vi "Write.vi"(8 "error in":errorcluster, 10 "CAN Message":T1 {"MSG type" format="%x"; "ID" format="%.0x"}, 11 "PCAN in":refnum<class "PCAN.lvclass">) -> (0 "error out":errorcluster, 3 "PCAN out":refnum<class "PCAN.lvclass">)   [LabVIEW 2025]
uses:
  PCAN.lvclass/PCAN.ctl
  D:/git/HAL/HAL/Configurations/CFG Base/CFG Base.lvclass
  PCAN.lvclass
  C:/Users/tupp_js/Documents/LabVIEW Data/HAL/source/Devices/PCAN/PCAN.lvclass
  C:/Users/tupp_js/Documents/LabVIEW Data/HAL/source/Interfaces/ICommunicate/ICommunicate.lvclass
  C:/Users/tupp_js/Documents/LabVIEW Data/HAL/source/Interfaces/IConfigurable/IConfigurable.lvclass
  C:/Users/tupp_js/Documents/LabVIEW Data/HAL/source/Interfaces/IConfigurableFromDBC/IConfigurableFromDBC.lvclass
  C:/Users/tupp_js/Documents/LabVIEW Data/HAL/source/Interfaces/IRunnable/IRunnable.lvclass
  C:/Users/tupp_js/Documents/LabVIEW Data/HAL/source/Interfaces/IConfigure/IConfigure.lvclass
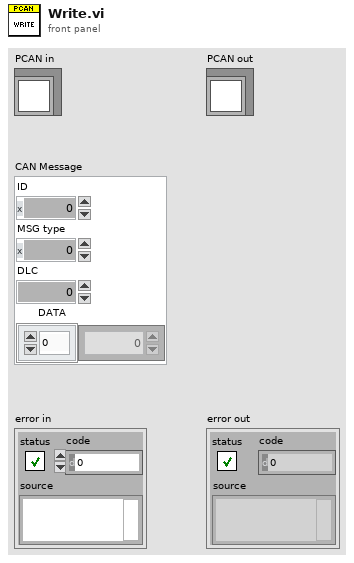
[diagram p1: front panel]
types:
  T1 = cluster{"ID":u32, "MSG type":u8, "DLC":u8, "DATA":u8[]}
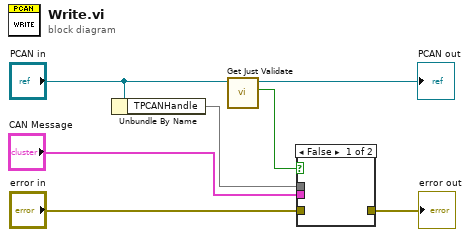
[diagram p0: block diagram]
diagram:
  n1 = Unbundle By Name("PCAN in") -> ("TPCANHandle"=w4)
  n2 = call "Get Just Validate.vi"("CFG Base in"="PCAN in") -> ("Just Validate"=w1:bool, "CFG Base out"=→"PCAN out":refnum<class "CFG Base.lvclass">)  [unwired: 9 in]
  n3 = case shown="False" w1 {
    tunnel: "error in" -> [_ w8]
    tunnel: [_ w8] -> w6
    tunnel: w4 -> [_ _]
    tunnel: "CAN Message" -> [_ _]
    frame False {
    }
    frame True {
    }
  }
  "error out" <- w6
